vi "转置数组.vi"() -> ()   [LabVIEW 2010]
panel:
  out "转置后的数组":i32[][](array[numeric])
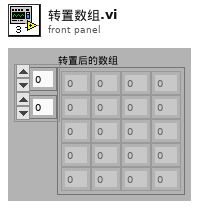
[diagram p1: front panel]
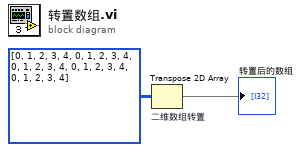
[diagram p0: block diagram]
diagram:
  n1 = Transpose 2D Array "二维数组转置"(2D array=i32[][] [[0, 1, 2, 3, 4], [0, 1, 2, 3, 4], [0, 1, 2, 3, 4], [0, 1, 2, 3, 4], [0, 1, 2, 3, 4]] ("Array")) -> (transposed array=→"转置后的数组":i32[][])
